vi "Query Number.vi"(8 "error in (no error)":errorcluster, 10 "Query String":string, 11 "BH Druck PACE Series in":refnum<class "BH Druck PACE Series.lvclass">) -> (0 "error out":errorcluster, 2 "Numeric Result":dbl, 3 "BH Druck PACE Series out":refnum<class "BH Druck PACE Series.lvclass">)   [LabVIEW 2022 SP3, in "BH Druck PACE Series.lvclass"]
uses:
  BH Druck PACE Series.lvclass
  BH Druck PACE Series.lvclass/BH Druck PACE Series.ctl
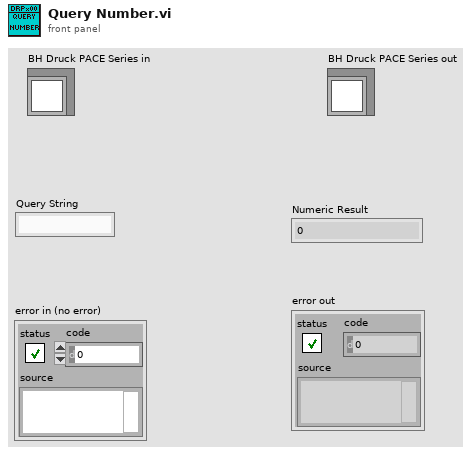
[diagram p1: front panel]
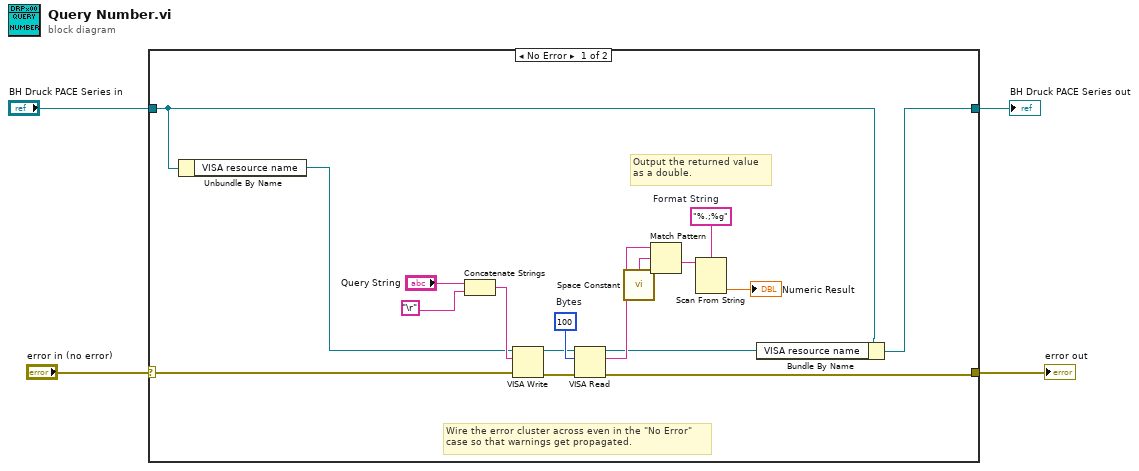
[diagram p0: block diagram]
diagram:
  n1 = case shown="No Error" "error in (no error)" {
    selector: "error in (no error)" -> [w10 w23]
    tunnel: [w9 w23] -> w3
    tunnel: [w5 w22] -> w1
    tunnel: "BH Druck PACE Series in" -> [w7 w22]
    frame No Error {
      w20 = "%.;%g"  # Format String
      w19 = u32 100  # Bytes
      # "Output the returned value\nas a double."
      # "Wire the error cluster across even in the \"No Error\"\ncase so that warnings get propagated."
      n2 = Unbundle By Name(w7) -> ("VISA resource name"=w8:refnum<visa-resource-name>)
      n3 = Concatenate Strings("Query String", "\r" ("Carriage Return Constant")) -> (w12:string)
      n4 = VISA Write(VISA resource name=w8, write buffer=w12, error in (no error)=w10) -> (VISA resource name out=w18:refnum<visa-resource-name>, error out=w17:errorcluster)  [unwired: 1 out]
      n5 = VISA Read(VISA resource name=w18, byte count=w19, error in (no error)=w17) -> (VISA resource name out=w6:refnum<visa-resource-name>, read buffer=w14:string, error out=w9:errorcluster)  [unwired: 1 out]
      n6 = call <vilib>:"Space Constant.vi"() -> ("String"=w16:string)
      n7 = Match Pattern(string=w14, regular expression=w16) -> (after substring=w15:string)  [unwired: 1 in, 3 out]
      n8 = Scan From String(format string=w20, input string=w15) -> (output 1=→"Numeric Result":dbl)  [unwired: 3 in, 3 out]
      n9 = Bundle By Name(cluster=w7, "VISA resource name"=w6) -> (w5:refnum<class "BH Druck PACE Series.lvclass">)
    }
    frame Error {
    }
  }
  "error out" <- w3
  "BH Druck PACE Series out" <- w1
